vi "UHR-Fleezers Control (host) - 11.9c.vi"() -> ()   [LabVIEW 2014] (continued)
        n1081 = xnode "Read/Write Control"("FPGA VI Reference In"=w1450, "error in"=w1448, "Operating Mode"=w1447, "Operating Mode 2"=w1447, "Green FB On/Off"=w1446, "Red operating mode"=w1442, "RI operating mode 2"=w1442) -> ("error out"=w1449:errorcluster)  [unwired: 1 out]
      }
      event "Green Laser ON/OFF": Value Change {
        n1082 = event-data() -> ()  [unwired: 7 out]
        n1083 = property on="Green ON/Interlacing" class="Bool (strict)"("Val(Sgnl)"="Green Laser ON/OFF") -> ()  [unwired: 2 in, 2 out]
      }
      event "Test ttrig": Value Change {
        n1084 = event-data() -> ()  [unwired: 7 out]
        n1085 = xnode "Read/Write Control"("FPGA VI Reference In"=w1467, "error in"=w1466, "TTrig?"=TRUE) -> ("error out"=w1465:errorcluster)  [unwired: 1 out]
      }
      event "Neg. TTrig FPGA": Value Change {
        n1086 = event-data() -> ()  [unwired: 7 out]
        n1087 = xnode "Read/Write Control"("FPGA VI Reference In"=w1471, "error in"=w1470, "TTrig Negate Pos"="Neg. TTrig FPGA") -> ()  [unwired: 2 out]
      }
      event "- phase (APD 1 Gate)", "+ phase (APD 1 Gate)": Value Change {
        n1088 = event-data() -> ()  [unwired: 7 out]
        n1089 = local read "Phase Adj. (APD 1 Gate)"() -> (w1472:i16)
        n1090 = Negate(x=w1472) -> (-x=w1480:i16)
        n1091 = Select(t=w1480, s="- phase (APD 1 Gate)", f=w1472) -> (s? t:f=w1479:i16)
        n1092 = Or(x="- phase (APD 1 Gate)", y="+ phase (APD 1 Gate)") -> (x .or. y?=w1475:bool)
        n1093 = xnode "Read/Write Control"("FPGA VI Reference In"=w1482, "error in"=w1481, "Phase count adjustment (APD 1 Gate)"=w1479) -> ("FPGA VI Reference Out"=w1477:T20, "error out"=w1478:errorcluster)
        n1094 = xnode "Read/Write Control"("FPGA VI Reference In"=w1477, "error in"=w1478, "+ phase (APD 1 Gate)"=w1475) -> ("error out"=w1476:errorcluster)  [unwired: 1 out]
      }
      event "+ phase (APD 2 Gate)", "- phase (APD 2 Gate)": Value Change {
        n1095 = event-data() -> ()  [unwired: 7 out]
        n1096 = local read "Phase Adj. (APD 2 Gate)"() -> (w1483:i16)
        n1097 = Negate(x=w1483) -> (-x=w1491:i16)
        n1098 = Select(t=w1491, s="- phase (APD 2 Gate)", f=w1483) -> (s? t:f=w1490:i16)
        n1099 = Or(x="- phase (APD 2 Gate)", y="+ phase (APD 2 Gate)") -> (x .or. y?=w1486:bool)
        n1100 = xnode "Read/Write Control"("FPGA VI Reference In"=w1493, "error in"=w1492, "Phase count adjustment (APD 2 Gate)"=w1490) -> ("FPGA VI Reference Out"=w1488:T20, "error out"=w1489:errorcluster)
        n1101 = xnode "Read/Write Control"("FPGA VI Reference In"=w1488, "error in"=w1489, "+ phase (APD 2 Gate)"=w1486) -> ("error out"=w1487:errorcluster)  [unwired: 1 out]
      }
      event "Phase Adj. (APD Acq)", "+ phase (APD Acq)", "- phase (APD Acq)": Value Change {
        n1102 = event-data() -> ()  [unwired: 7 out]
        n1103 = local read "Phase Adj. (APD Acq)"() -> (w1496:i16)
        n1104 = Negate(x=w1496) -> (-x=w1502:i16)
        n1105 = Select(t=w1502, s="+ phase (APD Acq)", f=w1496) -> (s? t:f=w1501:i16)
        n1106 = Or(x="+ phase (APD Acq)", y="- phase (APD Acq)") -> (x .or. y?=w1497:bool)
        n1107 = xnode "Read/Write Control"("FPGA VI Reference In"=w1504, "error in"=w1503, "Phase Count Adjustment (APD Acq)"=w1501) -> ("FPGA VI Reference Out"=w1499:T20, "error out"=w1500:errorcluster)
        n1108 = xnode "Read/Write Control"("FPGA VI Reference In"=w1499, "error in"=w1500, "+ phase (APD Acq)"=w1497) -> ("error out"=w1498:errorcluster)  [unwired: 1 out]
      }
      event "Phase adj. (GI)", "+ phase (GI)", "- phase (GI)", "+phase (RI)", "- phase (RI)", "Phase adj. (RI)": Value Change {
        n1109 = event-data() -> ()  [unwired: 7 out]
        n1110 = Negate(x="Phase adj. (GI)") -> (-x=w1519:i16)
        n1111 = Select(t=w1519, s="+ phase (GI)", f="Phase adj. (GI)") -> (s? t:f=w1518:i16)
        n1112 = Or(x="+ phase (GI)", y="- phase (GI)") -> (x .or. y?=w1514:bool)
        n1113 = Negate(x="Phase adj. (RI)") -> (-x=w1509:i16)
        n1114 = Select(t=w1509, s="+phase (RI)", f="Phase adj. (RI)") -> (s? t:f=w1506:i16)
        n1115 = Or(x="+phase (RI)", y="- phase (RI)") -> (x .or. y?=w1505:bool)
        n1116 = xnode "Read/Write Control"("FPGA VI Reference In"=w1521, "error in"=w1520, "Phase count adjustment (GI)"=w1518, "Phase count adjustment (RI)"=w1506) -> ("FPGA VI Reference Out"=w1516:T20, "error out"=w1517:errorcluster)
        n1117 = xnode "Read/Write Control"("FPGA VI Reference In"=w1516, "error in"=w1517, "+ phase (GI)"=w1514, "+ phase (RI)"=w1505) -> ("error out"=w1515:errorcluster)  [unwired: 1 out]
      }
      event "+ phase (GI) 2", "- phase (GI) 2": Value Change {
        n1118 = event-data() -> ()  [unwired: 7 out]
        n1119 = Negate(x="Phase adj. (GI) 2") -> (-x=w1530:i16)
        n1120 = Select(t=w1530, s="+ phase (GI) 2", f="Phase adj. (GI) 2") -> (s? t:f=w1529:i16)
        n1121 = Or(x="+ phase (GI) 2", y="- phase (GI) 2") -> (x .or. y?=w1525:bool)
        n1122 = xnode "Read/Write Control"("FPGA VI Reference In"=w1532, "error in"=w1531, "Phase count adjustment (GI) 2"=w1529) -> ("FPGA VI Reference Out"=w1527:T20, "error out"=w1528:errorcluster)
        n1123 = xnode "Read/Write Control"("FPGA VI Reference In"=w1527, "error in"=w1528, "+ phase (GI) 2"=w1525) -> ("error out"=w1526:errorcluster)  [unwired: 1 out]
      }
      event "Phase adj. (Green FB)", "- phase (Green FB)", "+ phase (Green FB)": Value Change {
        n1124 = event-data() -> ()  [unwired: 7 out]
        n1125 = Negate(x="Phase adj. (Green FB)") -> (-x=w1541:i16)
        n1126 = Select(t=w1541, s="+ phase (Green FB)", f="Phase adj. (Green FB)") -> (s? t:f=w1540:i16)
        n1127 = Or(x="+ phase (Green FB)", y="- phase (Green FB)") -> (x .or. y?=w1536:bool)
        n1128 = xnode "Read/Write Control"("FPGA VI Reference In"=w1543, "error in"=w1542, "Phase count adjustment (Green FB)"=w1540) -> ("FPGA VI Reference Out"=w1538:T20, "error out"=w1539:errorcluster)
        n1129 = xnode "Read/Write Control"("FPGA VI Reference In"=w1538, "error in"=w1539, "+ phase (Green FB)"=w1536) -> ("error out"=w1537:errorcluster)  [unwired: 1 out]
      }
      event "Invert APD Gate", "APD Gate ON Count", "APD Gate OFF Count", "APD Gate", "APD Integration Time (s)", "APD 1 AO Mult.", "APD 2 AO Mult.", "Duty frequency (ON 1/N cycles)": Value Change {
        n1130 = event-data() -> ()  [unwired: 7 out]
        n1131 = Add(x="Interlace ON count", y="Interlace OFF count") -> (x+y=w1547:u16)
        n1132 = Add(x="APD Gate ON Count", y="APD Gate OFF Count") -> (x+y=w1560:u16)
        n1133 = Multiply(x="Duty frequency (ON 1/N cycles)", y=w1547) -> (x*y=w1546:u16)
        "Green FB Count" <- w1546
        n1134 = Subtract(x=w1546, y="Interlace ON count") -> (x-y=w1544:u16)
        n1135 = Multiply(x=w1560, y="Duty frequency (ON 1/N cycles)") -> (x*y=w1559:u16)
        n1136 = Subtract(x=w1559, y="APD Gate ON Count") -> (x-y=w1558:u16)
        n1137 = local read "DMA Update Period (s)"() -> (w1561:dbl)
        n1138 = Multiply(x="APD Integration Time (s)", y=40000000.0) -> (x*y=w1566:dbl)
        n1139 = Reciprocal(x="APD Integration Time (s)") -> (1/x=→"APD Acq Rate (Hz)":dbl)
        n1140 = To Unsigned Long Integer(number=w1566) -> (unsigned 32bit integer=w1550:u32)
        "APD Int. Count" <- w1550
        n1141 = xnode "Read/Write Control"("FPGA VI Reference In"=w1570, "error in"=w1569, "Invert APD Gate"="Invert APD Gate", "APD Gate ON Count"="APD Gate ON Count", "APD Gate OFF Count"=w1558, "APD Acq Rate Count"=w1550, "APD Gate Operating Mode"="APD Gate", "APD 1 AO scale factor"="APD 1 AO Mult.", "APD 2 AO scale factor"="APD 2 AO Mult.", "Green interlace ON count"="Interlace ON count", "Green interlace OFF count"=w1544, "Green interlace ON count 2"="Interlace ON count", "Green interlace OFF count 2"=w1544, "Green FB Count"=w1546, "RI ON count"="Interlace ON count", "RI OFF count"=w1544) -> ("error out"=w1568:errorcluster)  [unwired: 1 out]
        n1142 = Divide(x=w1561, y="APD Integration Time (s)") -> (x/y=w1564:dbl)
        n1143 = Multiply(x=2.0, y=w1564) -> (x*y=w1563:dbl)
        n1144 = local write "APD Samples/FIFO Acq."(w1564) -> ()
        n1145 = local write "APD Elements/DMA read"(w1563) -> ()
      }
      event "Number of F/B Scans (AOD)", "Scan Speed (nm/s)", "Scan BD", "Initial D (MHz)", "Step Size (nm)", "Scan Range (nm)", "Wiggle amp 1 (units?)": Value Change {
        w1632 = 123.0  # AOM cal (nm/MHz)
        n1146 = event-data() -> ()  [unwired: 7 out]
        n1147 = local read "BD 1 Frequency 1 (MHz)"() -> (w1615:dbl)
        n1148 = local read "AOM X Cal (nm/MHz)"() -> (w1607:dbl)
        n1149 = local read "BD 2 Frequency 1 (MHz)"() -> (w1621:dbl)
        n1150 = local read "X RF Frequency Limits (MHz)"() -> (w1619:T17)
        n1151 = local read "Y RF Frequency Limits (MHz)"() -> (w1616:T17)
        n1152 = Negate(x="Scan Range (nm)") -> (-x=w1585:dbl)
        n1153 = Divide(x=w1585, y=w1607) -> (x/y=w1589:dbl)
        n1154 = Select(t=w1619, s="Scan BD", f=w1616) -> (s? t:f=w1618:T17)
        n1155 = Select(t=w1615, s="Scan BD", f=w1621) -> (s? t:f=w1620:dbl)
        n1156 = Unbundle By Name(w1618) -> ("Maximum"=w1627:dbl, "Minimum"=w1626:dbl)
        n1157 = Add(x=w1589, y=w1620) -> (x+y=w1624:dbl)
        n1158 = Divide(x=w1585, y="Step Size (nm)") -> (x/y=w1604:dbl)
        n1159 = Divide(x="Step Size (nm)", y=w1607) -> (x/y=w1613:dbl)
        n1160 = Absolute Value(x=w1604) -> (abs(x)=w1588:dbl)
        n1161 = Sign(1:w1585) -> (0:w1586:dbl)
        n1162 = In Range and Coerce(upper limit=w1627, x=w1624, lower limit=w1626) -> (coerced(x)=w1623:dbl, In Range?=w1625:bool)
        n1163 = To Unsigned Quad Integer(1:w1588) -> (0:w1603:u64)
        "Scan steps (AOD)" <- w1603
        n1164 = call "IR AOM freq to word.vi"("Frequency In (MHz)"=w1613) -> ("Frequency Word Out (double)"=w1610:dbl)
        n1165 = Multiply(x=w1586, y=w1610) -> (x*y=w1587:dbl)
        n1166 = Subtract(x=w1624, y=w1623) -> (x-y=w1622:dbl)
        n1167 = To Quad Integer(1:w1587) -> (0:w1609:i64)
        "Incr. int (AOD)" <- w1609
        n1168 = Subtract(x=w1589, y=w1622) -> (x-y=w1608:dbl)
        "Scan Range (MHz)" <- w1608
        n1169 = Select(t=w1589, s=w1625, f=w1608) -> (s? t:f=w1628:dbl)
        n1170 = Multiply(x=w1608, y=w1607) -> (x*y=w1606:dbl)
        n1171 = Decrement(x=w1603) -> (x-1=w1656:u64)
        n1172 = Negate(x=w1606) -> (-x=w1602:dbl)
        n1173 = local write "Scan Range (nm)"(w1602) -> ()
        n1174 = Divide(x=w1628, y=w1656) -> (x/y=w1612:dbl)
        "Scan Increment (MHz)" <- w1612
        n1175 = call "IR AOM freq to word.vi"("Frequency In (MHz)"=w1612) -> ("Frequency Word Out (double)"=w1611:dbl)
        n1176 = Divide(x="Step Size (nm)", y="Scan Speed (nm/s)") -> (x/y=w1599:dbl)
        n1177 = To Quad Integer(1:w1611) -> ()  [unwired: 1 out]
        n1178 = local read "Number Interlace Sets"() -> (w1583:u8)
        n1179 = local read "AI Count (ticks)"() -> (w1584:u32)
        n1180 = local read "Total Counts (ticks)"() -> (w1582:u32)
        n1181 = local read "# Samples/trap"() -> (w1614:u32)
        n1182 = Multiply(x=w1584, y=w1583) -> (x*y=w1581:u32)
        n1183 = Divide(x=w1582, y=w1581) -> (x/y=w1580:dbl)
        n1184 = Select(t=w1615, s="Scan BD", f=w1621) -> (s? t:f=w1653:dbl)
        "Initial freq. (MHz)" <- w1653
        n1185 = Add(x=w1628, y=w1653) -> (x+y=→"Final freq. (MHz)":dbl)
        n1186 = Divide(x=w1582, y=40000000.0) -> (x/y=w1598:dbl)
        n1187 = Divide(x=w1599, y=w1598) -> (x/y=w1597:dbl)
        n1188 = To Unsigned Quad Integer(1:w1597) -> (0:w1572:u64)
        n1189 = Quotient & Remainder(x=w1572, y=u64 2) -> (x-y*floor(x/y)=w1576:u64)  [unwired: 1 out]
        n1190 = Equal?(x=w1576, y=u64 0) -> (x = y?=w1574:bool)
        n1191 = Decrement(x=w1572) -> (x-1=w1573:u64)
        n1192 = Select(t=w1572, s=w1574, f=w1573) -> (s? t:f=w1571:u64)
        "Cycles/step (AOD)" <- w1571
        n1193 = xnode "Read/Write Control"("FPGA VI Reference In"=w1664, "error in"=w1663, "Scan steps"=w1603, "Number of scans"="Number of F/B Scans (AOD)", "Cycles per step"=w1571, "Scan freq.  increment"=w1609, "Scan BD"="Scan BD") -> ("error out"=w1662:errorcluster)  [unwired: 1 out]
        n1194 = Multiply(x=w1603, y=w1571) -> (x*y=w1657:u64)
        n1195 = Multiply(x=w1657, y=u64 2) -> (x*y=w1579:u64)
        n1196 = Multiply(x=w1580, y=w1579) -> (x*y=w1578:dbl)
        "Data points/scan (f/b)" <- w1578
        n1197 = Multiply(x=w1578, y="Number of F/B Scans (AOD)") -> (x*y=w1660:dbl)
        "Data points/scans" <- w1660
        n1198 = Divide(x=w1660, y=w1614) -> (x/y=→"N sets should be saved":dbl)
        n1199 = Multiply(x=w1657, y=w1598) -> (x*y=w1596:dbl)
        "Time/Scan (s) (AOD)" <- w1596
        n1200 = Select(t=w1628, s="Scan BD", f=0.0) -> (s? t:f=w1654:dbl)
        n1201 = Select(t=0.0, s="Scan BD", f=w1628) -> (s? t:f=w1650:dbl)
        n1202 = local read "BD 2 Frequency 2 (MHz)"() -> (w1646:dbl)
        n1203 = local read "BD 1 Frequency 2 (MHz)"() -> (w1649:dbl)
        n1204 = Add(x=w1650, y=w1621) -> (x+y=w1647:dbl)
        n1205 = Add(x=w1615, y=w1654) -> (x+y=w1648:dbl)
        n1206 = Multiply(x=w1596, y=2.0) -> (x*y=w1595:dbl)
        n1207 = Multiply(x=w1595, y="Number of F/B Scans (AOD)") -> (x*y=w1592:dbl)
        n1208 = Divide(x=w1592, y=60.0) -> (x/y=→"Time to Finish All (min)":dbl)
        n1209 = Add(x="Trap 2 Bead Size (nm)", y="Trap 1 Bead Size (nm)") -> (x+y=w1636:dbl)
        n1210 = Divide(x=w1636, y=2.0) -> (x/y=w1630:dbl)
        n1211 = Subtract(x=w1647, y=w1646) -> (x-y=w1644:dbl)
        n1212 = Subtract(x=w1648, y=w1649) -> (x-y=w1645:dbl)
        n1213 = local read "Initial D (MHz)"() -> (w1633:dbl)
        n1214 = Square(x=w1644) -> (x^2=w1643:dbl)
        n1215 = Square(x=w1645) -> (x^2=w1642:dbl)
        n1216 = Add(x=w1642, y=w1643) -> (x+y=w1641:dbl)
        n1217 = Square Root(x=w1641) -> (sqrt(x)=w1640:dbl)
        "Final D (MHz)" <- w1640
        n1218 = Multiply(x=w1632, y=w1640) -> (x*y=w1639:dbl)
        n1219 = Multiply(x=w1633, y=w1632) -> (x*y=w1631:dbl)
        n1220 = Subtract(x=w1631, y=w1630) -> (x-y=→"Initial sep (nm)":dbl)
        n1221 = Subtract(x=w1639, y=w1630) -> (x-y=→"Final sep (nm)":dbl)
      }
      event "Freq or Amp switch first", "Swap F1 and F2", "Freq switch delay", "Amp switch delay": Value Change {
        n1222 = event-data() -> ()  [unwired: 7 out]
        n1223 = local read "Freq or Amp switch first"() -> (w1665:bool)
        n1224 = local read "Amp switch delay"() -> (w1666:u16)
        n1225 = local read "Freq switch delay"() -> (w1668:u16)
        n1226 = local read "Swap F1 and F2"() -> (w1667:bool)
        n1227 = xnode "Read/Write Control"("FPGA VI Reference In"=w1671, "error in"=w1670, "Freq switch delay"=w1668, "Swap F1 and F2"=w1667, "Amp switch delay"=w1666, "Freq or Amp switch first"=w1665) -> ("error out"=w1669:errorcluster)  [unwired: 1 out]
      }
      event "Scan steps (MCL)", "Number of scans (MCL)", "Scan Range (V)\n(of steps)", "2D or 1D Scan", "N APD Samp/step", "Fast Scan Dir", "Continuous MCL Scanning", "Scan lines (y)": Value Change {
        w1673 = 32767.0 ("y")
        n1228 = event-data() -> ()  [unwired: 7 out]
        n1229 = Select(t="Scan lines (y)", s="2D or 1D Scan", f="Number of scans (MCL)") -> (s? t:f=w1678:u64)
        n1230 = Decrement(x="Scan steps (MCL)") -> (x-1=w1694:u64)
        n1231 = Divide(x="Scan Range (V)\n(of steps)", y=w1694) -> (x/y=w1693:dbl)
        "Desired Scan Incr (V)" <- w1693
        n1232 = local read "APD Integration Time (s)"() -> (w1686:dbl)
        n1233 = Multiply(x=w1693, y=w1673) -> (x*y=w1702:dbl)
        n1234 = Divide(x=w1702, y=10.0) -> (x/y=w1692:dbl)
        "Desired incr (int)" <- w1692
        n1235 = local read "Update Count (MCL)"() -> (w1698:u32)
        n1236 = Round Toward -Infinity(1:w1692) -> (0:w1701:dbl)
        n1237 = To Word Integer(number=w1701) -> (16bit integer=w1676:i16)
        "Actual Incr. int (MCL)" <- w1676
        n1238 = Multiply(x=w1686, y=40000000.0) -> (x*y=w1699:dbl)
        n1239 = Divide(x=w1699, y=w1698) -> (x/y=w1697:dbl)
        n1240 = Multiply(x=i16 10, y=w1676) -> (x*y=w1674:i16)
        n1241 = Multiply(x="N APD Samp/step", y=w1697) -> (x*y=w1696:dbl)
        "Cycles/step (MCL)" <- w1696
        n1242 = Divide(x=w1674, y=w1673) -> (x/y=→"Actual MCL Inc (V)":dbl)
        n1243 = Multiply(x="N APD Samp/step", y="Scan steps (MCL)") -> (x*y=w1688:dbl)
        n1244 = local read "APD Samples/FIFO Acq."() -> (w1685:dbl)
        n1245 = Multiply(x=w1688, y=u64 2) -> (x*y=w1687:dbl)
        "Data points/scan (f+b)" <- w1687
        n1246 = Multiply(x=w1687, y=w1678) -> (x*y=w1705:dbl)
        "Data points/scans (MCL)" <- w1705
        n1247 = Multiply(x=w1686, y=w1687) -> (x*y=w1679:dbl)
        "Time/f+b scan (s) (MCL)" <- w1679
        n1248 = Divide(x=w1705, y=w1685) -> (x/y=→"N sets should be saved (MCL)":dbl)
        n1249 = Multiply(x=w1679, y=w1678) -> (x*y=→"Total Time (s)":dbl)
        n1250 = Not(x="Fast Scan Dir") -> (.not. x?=w1683:bool)
        n1251 = xnode "Read/Write Control"("FPGA VI Reference In"=w1709, "error in"=w1708, "Scan steps (MCL)"="Scan steps (MCL)", "Number of scans (MCL)"=w1678, "Cycles per step (MCL)"=w1696, "Scan freq.  increment (MCL)"=w1676, "1D or 2D Scan?"="2D or 1D Scan", "MCL Scan Axis"=w1683, "Cont. Scan (MCL)"="Continuous MCL Scanning") -> ("error out"=w1707:errorcluster)  [unwired: 1 out]
      }
      event "Read Cal": Value Change {
        w1711 = 1000.0 ("y")
        n1252 = event-data() -> ()  [unwired: 7 out]
        n1253 = local read "Save file name"() -> (w1736:path)
        n1254 = local write "Read Cal"(FALSE ("Read Cal")) -> ()
        n1255 = Strip Path(path=w1736) -> (stripped path=w1735:path)  [unwired: 1 out]
        n1256 = Path To String(path=w1735) -> (string=w1734:string)
        n1257 = Concatenate Strings(w1734, "\\current.cal" ("string")) -> (w1732:string)
        n1258 = String To Path(string=w1732) -> (path=w1731:path)
        n1259 = Open/Create/Replace File(file path (use dialog)=w1731, operation (0:open)=T26."open", access (0:read/write)=enum16{"read/write", "read-only", "write-only"}."read-only") -> (refnum out=w1739:refnum<file>, error out=w1725:errorcluster)  [unwired: 1 in, 3 out]
        n1260 = Deny Access(4:w1725, 7:w1739) -> (0:w1724:errorcluster, 3:w1730:refnum<file>)  [unwired: 1 out]
        n1261 = Read from Binary File(5:0.0, 8:w1724, 9:T25."big-endian, network order" ("byte order (0:big-endian, network order)"), 10:-1 ("count (1)"), 11:w1730) -> (0:w1723:errorcluster, 2:w1721:dbl[], 3:w1726:refnum<file>)  [unwired: 2 out]
        n1262 = Array To Cluster(array=w1721) -> (cluster=w1720:T28)
        n1263 = Unbundle(w1720) -> ("[0]"=w1719:dbl, "[1]"=w1718:dbl, "[2]"=w1717:dbl, "[3]"=w1716:dbl, "[4]"=w1715:dbl, "[5]"=w1714:dbl)
        n1264 = Close File(refnum=w1726, error in=w1723) -> (error out=→"Read cal error":errorcluster)  [unwired: 1 out]
        n1265 = Multiply(x=w1714, y=w1711) -> (x*y=w1712:dbl)
        n1266 = local write "T2 k_x (pN/nm)"(w1716) -> ()
        n1267 = local write "T1 k_x (pN/nm)"(w1717) -> ()
        n1268 = local write "T1 a_x (nm/V)"(w1719) -> ()
        n1269 = local write "T2 a_x (nm/V)"(w1718) -> ()
        n1270 = Multiply(x=w1715, y=w1711) -> (x*y=w1713:dbl)
        n1271 = local write "T1 offset_x (mV)"(w1713) -> ()
        n1272 = local write "T2 offset_x (mV)"(w1712) -> ()
      }
      event "Read FX file": Value Change {
        n1273 = event-data() -> ()  [unwired: 7 out]
        n1274 = local write "Read FX file"(FALSE ("Read residual")) -> ()
        n1275 = local read "Save file name"() -> (w1764:path)
        n1276 = Strip Path(path=w1764) -> (stripped path=w1763:path)  [unwired: 1 out]
        n1277 = Path To String(path=w1763) -> (string=w1762:string)
        n1278 = Concatenate Strings(w1762, "\\current.cal" ("string")) -> (w1760:string)
        n1279 = String To Path(string=w1760) -> (path=w1759:path)
        n1280 = Open/Create/Replace File(file path (use dialog)=w1759, operation (0:open)=T26."open", access (0:read/write)=enum16{"read/write", "read-only", "write-only"}."read-only") -> (refnum out=w1756:refnum<file>, error out=w1753:errorcluster)  [unwired: 3 in, 1 out]
        n1281 = Deny Access(4:w1753, 7:w1756) -> (0:w1752:errorcluster, 3:w1755:refnum<file>)  [unwired: 1 in]
        n1282 = Read from Binary File(5:0.0, 8:w1752, 9:T25."big-endian, network order" ("byte order (0:big-endian, network order)"), 10:-1 ("count"), 11:w1755) -> (0:w1748:errorcluster, 2:w1742:dbl[], 3:w1749:refnum<file>)  [unwired: 1 in, 1 out]
        n1283 = Index Array(array=w1742, index=6) -> (element=→"Bad fit error":dbl)
        n1284 = Index Array(array=w1742, index=7) -> (element=→"Fit offset":dbl)
        n1285 = Index Array(array=w1742, index=8) -> (element=→"Hyst. error":dbl)
        n1286 = Close File(refnum=w1749, error in=w1748) -> ()  [unwired: 2 out]
      }
      event "Abort MCL Scan": Value Change {
        n1287 = event-data() -> ()  [unwired: 7 out]
        n1288 = local write "MCL Scanning"(FALSE ("MCL Scanning")) -> ()
        n1289 = xnode "Read/Write Control"("FPGA VI Reference In"=w1769, "error in"=w1768, "Abort scan (MCL)"="Abort MCL Scan") -> ("error out"=w1767:errorcluster)  [unwired: 1 out]
      }
      event "Update Count (MCL)": Value Change {
        n1290 = event-data() -> ()  [unwired: 7 out]
        n1291 = xnode "Read/Write Control"("FPGA VI Reference In"=w1773, "error in"=w1772, "MCL count"="Update Count (MCL)") -> ("error out"=w1771:errorcluster)  [unwired: 1 out]
      }
      event "Phase adjust (MCL)", "+ phase (MCL)", "- phase (MCL)": Value Change {
        n1292 = event-data() -> ()  [unwired: 7 out]
        n1293 = Negate(x="Phase adjust (MCL)") -> (-x=w1782:i16)
        n1294 = Select(t=w1782, s="- phase (MCL)", f="Phase adjust (MCL)") -> (s? t:f=w1780:i16)
        n1295 = Or(x="- phase (MCL)", y="+ phase (MCL)") -> (x .or. y?=w1775:bool)
        n1296 = xnode "Read/Write Control"("FPGA VI Reference In"=w1784, "error in"=w1783, "Phase count adjustment (MCL)"=w1780) -> ("FPGA VI Reference Out"=w1776:T20, "error out"=w1777:errorcluster)
        n1297 = xnode "Read/Write Control"("FPGA VI Reference In"=w1776, "error in"=w1777, "+ phase (MCL)"=w1775) -> ("error out"=w1774:errorcluster)  [unwired: 1 out]
      }
      event "Abort AOD Scan": Value Change {
        n1298 = event-data() -> ()  [unwired: 7 out]
        n1299 = xnode "Read/Write Control"("FPGA VI Reference In"=w1788, "error in"=w1787, "Abort scan"="Abort AOD Scan") -> ("error out"=w1786:errorcluster)  [unwired: 1 out]
      }
      event "Continuous AOD Scanning": Value Change {
        n1300 = event-data() -> ()  [unwired: 7 out]
        n1301 = xnode "Read/Write Control"("FPGA VI Reference In"=w1792, "error in"=w1791, "Cont. Scan"="Continuous AOD Scanning") -> ("error out"=w1790:errorcluster)  [unwired: 1 out]
      }
      event "Index": Value Change {
        n1302 = event-data() -> ()  [unwired: 7 out]
        n1303 = call "Create new save file.vi"("Insert"="", "Ext"=".dat" ("string"), "Index In"="Index") -> ("Path Out"=→"Save file name":path, "Index Out"=w1793:dbl)
        "Save index" <- w1793
        n1304 = local write "Index"(w1793) -> ()
      }
      event "AO1", "AO2": Value Change {
        w1808 = 10.0 ("y")
        w1807 = 32767.0 ("y")
        n1305 = event-data() -> ()  [unwired: 7 out]
        n1306 = local read "AO2"() -> (w1806:dbl)
        n1307 = local read "AO1"() -> (w1803:dbl)
        n1308 = Multiply(x=w1803, y=w1807) -> (x*y=w1802:dbl)
        n1309 = Multiply(x=w1806, y=w1807) -> (x*y=w1805:dbl)
        n1310 = Divide(x=w1802, y=w1808) -> (x/y=w1801:dbl)
        n1311 = Divide(x=w1805, y=w1808) -> (x/y=w1804:dbl)
        n1312 = To Word Integer(number=w1801) -> (16bit integer=w1809:i16)
        n1313 = To Word Integer(number=w1804) -> (16bit integer=w1810:i16)
        n1314 = xnode "Read/Write Control"("FPGA VI Reference In"=w1800, "error in"=w1799, "AO1"=w1809, "AO2"=w1810) -> ("error out"=w1798:errorcluster)  [unwired: 1 out]
      }
      event "Inject Pump 1": Value Change {
        n1315 = event-data() -> ()  [unwired: 7 out]
        n1316 = local read "Use Harvard pumps\nfor beads (else Chemyx)"() -> (w1812:bool)
        n1317 = case shown="True" w1812 {
          tunnel: "Inject Pump 1" -> [w1816 w1854]
          tunnel: w1811 -> [_ w1855]
          frame False {
            n1318 = local read "Pump write delay (ms)"() -> (w1815:dbl)
            n1319 = local read "Chemyx Syringe Pump Serial Port"() -> (w1814:refnum<visa-resource-name>)
            n1320 = case shown="True" w1816 {
              tunnel: w1815 -> [w1822 w1836]
              tunnel: w1814 -> [w1819 w1835]
              frame False {
                n1321 = flat-sequence {
                  tunnel: w1819 -> [w1823]
                  tunnel: [w1823] -> w1820
                  tunnel: w1822 -> [_]
                  tunnel: [w1826] -> w1821
                  tunnel: w1820 -> [w1826]
                  tunnel: w1821 -> [w1827]
                  tunnel: [w1827] -> w1817
                  tunnel: [w1829] -> w1818
                  tunnel: w1817 -> [w1829]
                  tunnel: w1818 -> [w1831]
                  frame #0 {
                    n1322 = call "Write to pump.vi"("string"="enter pump1", "VISA resource name"=w1823) -> ()  [unwired: 1 out]
                  }
                  frame #1 {
                    n1323 = Wait (ms)(milliseconds to wait="Pump pause delay (ms)") -> ()  [unwired: 1 out]
                  }
                  frame #2 {
                    n1324 = call "Write to pump.vi"("string"="stop", "VISA resource name"=w1827) -> ()  [unwired: 1 out]
                  }
                  frame #3 {
                    n1325 = Wait (ms)(milliseconds to wait=u32 500) -> ()  [unwired: 1 out]
                  }
                  frame #4 {
                    n1326 = call "Write to pump.vi"("string"="stop", "VISA resource name"=w1831) -> ()  [unwired: 1 out]
                  }
                }
              }
              frame True {
                n1327 = flat-sequence {
                  tunnel: w1835 -> [w1845]
                  tunnel: w1836 -> [w1840]
                  tunnel: w1836 -> [w1847]
                  tunnel: w1835 -> [w1848]
                  tunnel: [w1848] -> w1833
                  tunnel: [w1850] -> w1834
                  tunnel: w1833 -> [w1850]
                  tunnel: w1834 -> [w1852]
                  frame #0 {
                    n1328 = local read "All Pump Parameters"() -> (w1839:T5)
                    n1329 = Unbundle By Name(w1839) -> ("Pump 1"=w1846:T29)
                    n1330 = call "Set pump parameters.vi"("Pump write delay (ms)"=w1840, "Volume (uL)"="Ch 1 Inject Volume (uL)", "Rate (uL/h)"="Ch 1 Inject Rate (ul/h)", "Units"=4.0, "Pump #"=1.0, "Pump Parameters In"=w1846, "VISA resource name"=w1845) -> ("Pump Parameters Out"=w1838:T29)  [unwired: 3 in]
                    n1331 = Bundle By Name(cluster=w1839, "Pump 1"=w1838) -> (w1837:T5)
                    n1332 = local write "All Pump Parameters"(w1837) -> ()
                  }
                  frame #1 {
                    n1333 = Wait (ms)(milliseconds to wait=w1847) -> ()  [unwired: 1 out]
                  }
                  frame #2 {
                    n1334 = call "Write to pump.vi"("string"="start", "VISA resource name"=w1848) -> ()  [unwired: 1 out]
                  }
                  frame #3 {
                    n1335 = Wait (ms)(milliseconds to wait=u32 500) -> ()  [unwired: 1 out]
                  }
                  frame #4 {
                    n1336 = call "Write to pump.vi"("string"="start", "VISA resource name"=w1852) -> ()  [unwired: 1 out]
                  }
                }
              }
            }
          }
          frame True {
            n1337 = case shown="True" w1854 {
              tunnel: w1855 -> [w1856 w1866]
              frame False {
                n1338 = flat-sequence {
                  tunnel: w1856 -> [w1858]
                  frame #0 {
                    n1339 = local write "Flushing P1"(FALSE ("Flushing P1")) -> ()
                    n1340 = Concatenate Strings("stop" ("string"), "\r") -> (w1860:string)
                    n1341 = VISA Write(VISA resource name=w1858, write buffer=w1860) -> ()  [unwired: 1 in, 3 out]
                  }
                  frame #1 {
                    n1342 = property on="Clear Volume P1" class="Bool (strict)"("Val(Sgnl)"=TRUE ("Value (Signaling)")) -> ()  [unwired: 2 in, 2 out]
                  }
                }
              }
              frame True {
                n1343 = local read "Normal Flow Rate (ul/h) P1"() -> (w1864:dbl)
                n1344 = Number To Decimal String(number=w1864) -> (decimal integer string=w1870:string)  [unwired: 1 in]
                n1345 = Concatenate Strings("irate  " ("string"), w1870, " u/h" ("string"), "\r") -> (w1868:string)
                n1346 = VISA Write(VISA resource name=w1866, write buffer=w1868) -> (VISA resource name out=w1865:refnum<visa-resource-name>)  [unwired: 1 in, 2 out]
                n1347 = Concatenate Strings("irun" ("string"), "\r") -> (w1872:string)
                n1348 = VISA Write(VISA resource name=w1865, write buffer=w1872) -> ()  [unwired: 1 in, 3 out]
              }
            }
          }
        }
      }
      event "Inject Pump 3": Value Change {
        n1349 = event-data() -> ()  [unwired: 7 out]
        n1350 = local read "Use Harvard pumps\nfor beads (else Chemyx)"() -> (w1875:bool)
        n1351 = case shown="True" w1875 {
          tunnel: "Inject Pump 3" -> [w1879 w1918]
          tunnel: w1874 -> [_ w1917]
          frame False {
            n1352 = local read "Pump write delay (ms)"() -> (w1878:dbl)
            n1353 = case shown="True" w1879 {
              tunnel: w1878 -> [w1885 w1899]
              tunnel: "Chemyx Syringe Pump Serial Port" -> [w1882 w1898]
              frame False {
                n1354 = flat-sequence {
                  tunnel: w1882 -> [w1886]
                  tunnel: [w1886] -> w1883
                  tunnel: w1885 -> [_]
                  tunnel: [w1889] -> w1884
                  tunnel: w1883 -> [w1889]
                  tunnel: w1884 -> [w1890]
                  tunnel: [w1890] -> w1880
                  tunnel: [w1892] -> w1881
                  tunnel: w1880 -> [w1892]
                  tunnel: w1881 -> [w1894]
                  frame #0 {
                    n1355 = call "Write to pump.vi"("string"="enter pump3", "VISA resource name"=w1886) -> ()  [unwired: 1 out]
                  }
                  frame #1 {
                    n1356 = local read "Pump pause delay (ms)"() -> (w1888:u32)
                    n1357 = Wait (ms)(milliseconds to wait=w1888) -> ()  [unwired: 1 out]
                  }
                  frame #2 {
                    n1358 = call "Write to pump.vi"("string"="stop", "VISA resource name"=w1890) -> ()  [unwired: 1 out]
                  }
                  frame #3 {
                    n1359 = Wait (ms)(milliseconds to wait=u32 0) -> ()  [unwired: 1 out]
                  }
                  frame #4 {
                    n1360 = call "Write to pump.vi"("string"="stop", "VISA resource name"=w1894) -> ()  [unwired: 1 out]
                  }
                }
              }
              frame True {
                n1361 = flat-sequence {
                  tunnel: w1898 -> [w1908]
                  tunnel: w1899 -> [w1903]
                  tunnel: w1899 -> [w1910]
                  tunnel: w1898 -> [w1911]
                  tunnel: [w1911] -> w1897
                  tunnel: [w1914] -> w1896
                  tunnel: w1897 -> [w1914]
                  tunnel: w1896 -> [w1915]
                  frame #0 {
                    n1362 = local read "All Pump Parameters"() -> (w1902:T5)
                    n1363 = Unbundle By Name(w1902) -> ("Pump 3"=w1909:T29)
                    n1364 = call "Set pump parameters.vi"("Pump write delay (ms)"=w1903, "Volume (uL)"="Ch 3 Inject Volume (uL)", "Rate (uL/h)"="Ch 3 Inject Rate (ul/h)", "Units"=4.0, "Pump #"=3.0, "Pump Parameters In"=w1909, "VISA resource name"=w1908) -> ("Pump Parameters Out"=w1901:T29)  [unwired: 3 in]
                    n1365 = Bundle By Name(cluster=w1902, "Pump 3"=w1901) -> (w1900:T5)
                    n1366 = local write "All Pump Parameters"(w1900) -> ()
                  }
                  frame #1 {
                    n1367 = Wait (ms)(milliseconds to wait=w1910) -> ()  [unwired: 1 out]
                  }
                  frame #2 {
                    n1368 = call "Write to pump.vi"("string"="start", "VISA resource name"=w1911) -> ()  [unwired: 1 out]
                  }
                  frame #3 {
                    n1369 = Wait (ms)(milliseconds to wait=u32 500) -> ()  [unwired: 1 out]
                  }
                  frame #4 {
                    n1370 = call "Write to pump.vi"("string"="start", "VISA resource name"=w1915) -> ()  [unwired: 1 out]
                  }
                }
              }
            }
          }
          frame True {
            n1371 = case shown="True" w1918 {
              tunnel: w1917 -> [w1919 w1926]
              frame False {
                n1372 = flat-sequence {
                  tunnel: w1919 -> [w1921]
                  frame #0 {
                    n1373 = local write "Flushing P3"(FALSE ("Flushing P3")) -> ()
                    n1374 = Concatenate Strings("stop" ("string"), "\r") -> (w1923:string)
                    n1375 = VISA Write(VISA resource name=w1921, write buffer=w1923) -> ()  [unwired: 1 in, 3 out]
                  }
                  frame #1 {
                    n1376 = property on="Clear Volume P3" class="Bool (strict)"("Val(Sgnl)"=TRUE ("Value (Signaling)")) -> ()  [unwired: 2 in, 2 out]
                  }
                }
              }
              frame True {
                n1377 = local read "Normal Flow Rate (ul/h) P3"() -> (w1927:dbl)
                n1378 = Number To Decimal String(number=w1927) -> (decimal integer string=w1933:string)  [unwired: 1 in]
                n1379 = Concatenate Strings("irate  " ("string"), w1933, " u/h" ("string"), "\r") -> (w1931:string)
                n1380 = VISA Write(VISA resource name=w1926, write buffer=w1931) -> (VISA resource name out=w1929:refnum<visa-resource-name>)  [unwired: 1 in, 2 out]
                n1381 = Concatenate Strings("irun" ("string"), "\r") -> (w1935:string)
                n1382 = VISA Write(VISA resource name=w1929, write buffer=w1935) -> ()  [unwired: 1 in, 3 out]
              }
            }
          }
        }
      }
      event "Inject Pump 2": Value Change {
        n1383 = event-data() -> ()  [unwired: 7 out]
        n1384 = local read "Pump write delay (ms)"() -> (w1939:dbl)
        n1385 = local read "Chemyx Syringe Pump Serial Port"() -> (w1937:refnum<visa-resource-name>)
        n1386 = flat-sequence {
          tunnel: w1937 -> [w1952]
          tunnel: w1939 -> [w1948]
          tunnel: "Inject Pump 2" -> [_]
          tunnel: w1939 -> [w1954]
          tunnel: w1937 -> [w1955]
          frame #0 {
            n1387 = local read "All Pump Parameters"() -> (w1947:T5)
            n1388 = Multiply(x=60.0, y="Flush Center Ch Rate (ul/m)") -> (x*y=w1944:dbl)
            n1389 = Unbundle By Name(w1947) -> ("Pump 2"=w1953:T29)
            n1390 = call "Set pump parameters.vi"("Pump write delay (ms)"=w1948, "Volume (uL)"="Flush Center Ch Volume (uL)", "Rate (uL/h)"=w1944, "Units"=3.0, "Pump #"=2.0, "Pump Parameters In"=w1953, "VISA resource name"=w1952) -> ("Pump Parameters Out"=w1946:T29)  [unwired: 3 in]
            n1391 = Bundle By Name(cluster=w1947, "Pump 2"=w1946) -> (w1945:T5)
            n1392 = Add(x="Flush Center Ch Volume (uL)", y="Total Volume\nFlushed (uL)") -> (x+y=w1941:dbl)
            n1393 = local write "All Pump Parameters"(w1945) -> ()
            n1394 = local write "Total Volume\nFlushed (uL)"(w1941) -> ()
          }
          frame #1 {
            n1395 = Wait (ms)(milliseconds to wait=w1954) -> ()  [unwired: 1 out]
          }
          frame #2 {
            n1396 = call "Write to pump.vi"("string"="start", "VISA resource name"=w1955) -> ()  [unwired: 1 out]
          }
        }
      }
      event "Sample Channel\nFlow": Value Change {
        n1397 = event-data() -> ()  [unwired: 7 out]
        n1398 = case shown="True" "Sample Channel\nFlow" {
          tunnel: w1958 -> [w1959 w1965]
          frame False {
            n1399 = flat-sequence {
              tunnel: w1959 -> [w1961]
              frame #0 {
                n1400 = local write "Flushing samp"(FALSE ("Flushing samp")) -> ()
                n1401 = Concatenate Strings("stop" ("string"), "\r") -> (w1964:string)
                n1402 = VISA Write(VISA resource name=w1961, write buffer=w1964) -> ()  [unwired: 1 in, 3 out]
              }
            }
          }
          frame True {
            n1403 = local read "Normal Flow rate (mL/h)"() -> (w1975:dbl)
            n1404 = Number To Decimal String(number=w1975) -> (decimal integer string=w1974:string)  [unwired: 1 in]
            n1405 = Concatenate Strings("irate " ("string"), w1974, " u/h" ("string"), "\r") -> (w1970:string)
            n1406 = VISA Write(VISA resource name=w1965, write buffer=w1970) -> (VISA resource name out=w1969:refnum<visa-resource-name>)  [unwired: 1 in, 2 out]
            n1407 = Concatenate Strings("irun" ("string"), "\r") -> (w1966:string)
            n1408 = VISA Write(VISA resource name=w1969, write buffer=w1966) -> ()  [unwired: 1 in, 3 out]
          }
        }
      }
      event "Start Flow": Value Change {
        n1409 = event-data() -> ()  [unwired: 7 out]
        n1410 = local write "Sample Channel\nFlow"(TRUE ("Sample Channel\nFlow")) -> ()
        n1411 = local write "Start Flow"(FALSE ("Start Flow")) -> ()
        n1412 = Concatenate Strings("irun" ("string"), "\r") -> (w1980:string)
        n1413 = VISA Write(VISA resource name=w1976, write buffer=w1980) -> ()  [unwired: 1 in, 3 out]
      }
      event "Stop Flow": Value Change {
        w1982 = FALSE ("Stop Flow")
        n1414 = event-data() -> ()  [unwired: 7 out]
        n1415 = local write "Stop Flow"(w1982) -> ()
        n1416 = local write "Sample Channel\nFlow"(w1982) -> ()
        n1417 = Concatenate Strings("stop" ("string"), "\r") -> (w1985:string)
        n1418 = VISA Write(VISA resource name=w1983, write buffer=w1985) -> ()  [unwired: 1 in, 3 out]
      }
      event "Normal Flow rate (mL/h)": Value Change {
        n1419 = event-data() -> ()  [unwired: 7 out]
        n1420 = Number To Decimal String(number="Normal Flow rate (mL/h)") -> (decimal integer string=w1992:string)  [unwired: 1 in]
        n1421 = Concatenate Strings("irate  " ("string"), w1992, " u/h" ("string"), "\r") -> (w1991:string)
        n1422 = VISA Write(VISA resource name=w1988, write buffer=w1991) -> ()  [unwired: 1 in, 3 out]
      }
      event "Flush Sample": Value Change {
        n1423 = event-data() -> ()  [unwired: 7 out]
        n1424 = flat-sequence {
          tunnel: w1994 -> [w2022]
          frame #0 {
            # "set parameters (rate, volume) for flush, clear volume"
            n1425 = Number To Decimal String(number="Flush rate (mL/m)") -> (decimal integer string=w2018:string)  [unwired: 1 in]
            n1426 = local write "Sample Channel\nFlow"(TRUE ("Sample Channel\nFlow")) -> ()
            n1427 = Concatenate Strings("irate  " ("string"), w2018, " u/m" ("string"), "\r") -> (w2020:string)
            n1428 = VISA Write(VISA resource name=w2022, write buffer=w2020) -> (VISA resource name out=w2016:refnum<visa-resource-name>)  [unwired: 1 in, 2 out]
            n1429 = Number To Decimal String(number="Flush volume (mL)") -> (decimal integer string=w2007:string)  [unwired: 1 in]
            n1430 = Reciprocal(x="Flush rate (mL/m)") -> (1/x=w2001:dbl)
            n1431 = Concatenate Strings("tvolume  " ("string"), w2007, " u" ("string"), "\r") -> (w2005:string)
            n1432 = Multiply(x=w2001, y="Flush volume (mL)") -> (x*y=w1999:dbl)
            n1433 = VISA Write(VISA resource name=w2016, write buffer=w2005) -> (VISA resource name out=w2004:refnum<visa-resource-name>)  [unwired: 1 in, 2 out]
            n1434 = Multiply(x=w1999, y=60.0) -> (x*y=→"Samp Flush Time (s)":dbl)
            n1435 = Concatenate Strings("cvolume" ("string"), "\r") -> (w2003:string)
            n1436 = VISA Write(VISA resource name=w2004, write buffer=w2003) -> (VISA resource name out=w2014:refnum<visa-resource-name>)  [unwired: 1 in, 2 out]
            n1437 = Concatenate Strings("irun" ("string"), "\r") -> (w2012:string)
            n1438 = VISA Write(VISA resource name=w2014, write buffer=w2012) -> ()  [unwired: 1 in, 3 out]
          }
          frame #1 {
            "Flushing samp" <- TRUE ("Boolean")
          }
        }
      }
      event "Flush Pump 3": Value Change {
        n1439 = event-data() -> ()  [unwired: 7 out]
        n1440 = flat-sequence {
          tunnel: w2024 -> [w2027]
          frame #0 {
            # "set paramaters (rate, volume) for flush, clear volume"
            n1441 = Number To Decimal String(number="Flush rate (uL/m) P3") -> (decimal integer string=w2049:string)  [unwired: 1 in]
            n1442 = local write "Inject Pump 3"(TRUE ("Inject Pump 3")) -> ()
            n1443 = Concatenate Strings("irate  " ("string"), w2049, " u/m" ("string"), "\r") -> (w2051:string)
            n1444 = VISA Write(VISA resource name=w2027, write buffer=w2051) -> (VISA resource name out=w2047:refnum<visa-resource-name>)  [unwired: 1 in, 2 out]
            n1445 = Reciprocal(x="Flush rate (uL/m) P3") -> (1/x=w2031:dbl)
            n1446 = Number To Decimal String(number="Volume (uL) P3") -> (decimal integer string=w2038:string)  [unwired: 1 in]
            n1447 = Multiply(x="Volume (uL) P3", y=w2031) -> (x*y=w2030:dbl)
            n1448 = Concatenate Strings("tvolume  " ("string"), w2038, " u" ("string"), "\r") -> (w2036:string)
            n1449 = Multiply(x=w2030, y=60.0) -> (x*y=→"HP3 Flush Time (s)":dbl)
            n1450 = VISA Write(VISA resource name=w2047, write buffer=w2036) -> (VISA resource name out=w2035:refnum<visa-resource-name>)  [unwired: 1 in, 2 out]
            n1451 = Concatenate Strings("cvolume" ("string"), "\r") -> (w2034:string)
            n1452 = VISA Write(VISA resource name=w2035, write buffer=w2034) -> (VISA resource name out=w2045:refnum<visa-resource-name>)  [unwired: 1 in, 2 out]
            n1453 = Concatenate Strings("irun" ("string"), "\r") -> (w2043:string)
            n1454 = VISA Write(VISA resource name=w2045, write buffer=w2043) -> ()  [unwired: 1 in, 3 out]
          }
          frame #1 {
            "Flushing P3" <- TRUE ("Flushing P3")
          }
        }
      }
      event "Flush Pump 1": Value Change {
        n1455 = event-data() -> ()  [unwired: 7 out]
        n1456 = flat-sequence {
          tunnel: [w2065] -> w2055
          tunnel: w2054 -> [w2058]
          tunnel: w2055 -> [_]
          frame #0 {
            # "set paramaters (rate, volume) for flush, clear volume"
            n1457 = local write "Inject Pump 1"(TRUE ("Inject Pump 1")) -> ()
            n1458 = Number To Decimal String(number="Flush rate (uL/m) P1") -> (decimal integer string=w2081:string)  [unwired: 1 in]
            n1459 = Concatenate Strings("irate  " ("string"), w2081, " u/m" ("string"), "\r") -> (w2083:string)
            n1460 = VISA Write(VISA resource name=w2058, write buffer=w2083) -> (VISA resource name out=w2079:refnum<visa-resource-name>)  [unwired: 1 in, 2 out]
            n1461 = Reciprocal(x="Flush rate (uL/m) P1") -> (1/x=w2062:dbl)
            n1462 = Number To Decimal String(number="Volume (uL) P1") -> (decimal integer string=w2070:string)  [unwired: 1 in]
            n1463 = Multiply(x="Volume (uL) P1", y=w2062) -> (x*y=w2061:dbl)
            n1464 = Concatenate Strings("tvolume  " ("string"), w2070, " u" ("string"), "\r") -> (w2068:string)
            n1465 = Multiply(x=w2061, y=60.0) -> (x*y=→"HP1 Flush Time (s)":dbl)
            n1466 = VISA Write(VISA resource name=w2079, write buffer=w2068) -> (VISA resource name out=w2067:refnum<visa-resource-name>)  [unwired: 1 in, 2 out]
            n1467 = Concatenate Strings("cvolume" ("string"), "\r") -> (w2066:string)
            n1468 = VISA Write(VISA resource name=w2067, write buffer=w2066) -> (VISA resource name out=w2077:refnum<visa-resource-name>)  [unwired: 1 in, 2 out]
            n1469 = Concatenate Strings("irun" ("string"), "\r") -> (w2075:string)
            n1470 = VISA Write(VISA resource name=w2077, write buffer=w2075) -> (VISA resource name out=w2065:refnum<visa-resource-name>)  [unwired: 1 in, 2 out]
          }
          frame #1 {
            "Flushing P1" <- TRUE ("Flushing P3")
          }
        }
      }
      event "Clear Volume": Value Change {
        n1471 = event-data() -> ()  [unwired: 7 out]
        n1472 = Number To Decimal String(number="Normal volume (mL)") -> (decimal integer string=w2090:string)  [unwired: 1 in]
        n1473 = Concatenate Strings("tvolume " ("string"), w2090, " u" ("string"), "\r") -> (w2087:string)
        n1474 = VISA Write(VISA resource name=w2093, write buffer=w2087) -> (VISA resource name out=w2086:refnum<visa-resource-name>)  [unwired: 1 in, 2 out]
        n1475 = local write "Clear Volume"(FALSE ("Clear Volume")) -> ()
        n1476 = Concatenate Strings("cvolume" ("string"), "\r") -> (w2095:string)
        n1477 = VISA Write(VISA resource name=w2086, write buffer=w2095) -> ()  [unwired: 1 in, 3 out]
      }
      event "Clear Volume P3": Value Change {
        n1478 = event-data() -> ()  [unwired: 7 out]
        n1479 = Concatenate Strings("cvolume" ("string"), "\r") -> (w2101:string)
        n1480 = VISA Write(VISA resource name=w2100, write buffer=w2101) -> ()  [unwired: 1 in, 3 out]
        n1481 = local write "Clear Volume P3"(FALSE ("Clear Volume P3")) -> ()
      }
      event "Clear Volume P1": Value Change {
        n1482 = event-data() -> ()  [unwired: 7 out]
        n1483 = Concatenate Strings("cvolume" ("string"), "\r") -> (w2106:string)
        n1484 = local write "Clear Volume P1"(FALSE ("Clear Volume P1")) -> ()
        n1485 = VISA Write(VISA resource name=w2105, write buffer=w2106) -> ()  [unwired: 1 in, 3 out]
      }
      event "Display On P3": Value Change {
        n1486 = event-data() -> ()  [unwired: 7 out]
        n1487 = Select(t="dim 100", s="Display On P3", f="dim 0") -> (s? t:f=w2112:string)
        n1488 = Concatenate Strings(w2112, "\r") -> (w2114:string)
        n1489 = VISA Write(VISA resource name=w2109, write buffer=w2114) -> ()  [unwired: 1 in, 3 out]
      }
      event "Display On P1": Value Change {
        n1490 = event-data() -> ()  [unwired: 7 out]
        n1491 = Select(t="dim 100", s="Display On P1", f="dim 0") -> (s? t:f=w2119:string)
        n1492 = Concatenate Strings(w2119, "\r") -> (w2121:string)
        n1493 = VISA Write(VISA resource name=w2116, write buffer=w2121) -> ()  [unwired: 1 in, 3 out]
      }
      event "Retract Pump 3": Value Change {
        n1494 = event-data() -> ()  [unwired: 7 out]
        n1495 = local write "Retract Pump 3"(FALSE ("Retract Pump 3")) -> ()
        n1496 = case shown="True" "Retract Pump 3" {
          tunnel: w2123 -> [_ w2126]
          frame False {
          }
          frame True {
            n1497 = Number To Decimal String(number="Retract Rate (mL/m)") -> (decimal integer string=w2144:string)  [unwired: 1 in]
            n1498 = Concatenate Strings("wrate  " ("string"), w2144, " u/m" ("string"), "\r") -> (w2146:string)
            n1499 = VISA Write(VISA resource name=w2126, write buffer=w2146) -> (VISA resource name out=w2137:refnum<visa-resource-name>)  [unwired: 1 in, 2 out]
            n1500 = Number To Decimal String(number="Retract Vol 3 (uL)") -> (decimal integer string=w2139:string)  [unwired: 1 in]
            n1501 = Concatenate Strings("tvolume  " ("string"), w2139, " u" ("string"), "\r") -> (w2136:string)
            n1502 = VISA Write(VISA resource name=w2137, write buffer=w2136) -> (VISA resource name out=w2132:refnum<visa-resource-name>)  [unwired: 1 in, 2 out]
            n1503 = Concatenate Strings("cvolume" ("string"), "\r") -> (w2133:string)
            n1504 = VISA Write(VISA resource name=w2132, write buffer=w2133) -> (VISA resource name out=w2127:refnum<visa-resource-name>)  [unwired: 1 in, 2 out]
            n1505 = Concatenate Strings("wrun" ("string"), "\r") -> (w2128:string)
            n1506 = VISA Write(VISA resource name=w2127, write buffer=w2128) -> ()  [unwired: 1 in, 3 out]
          }
        }
      }
      event "Retract Pump 1": Value Change {
        n1507 = event-data() -> ()  [unwired: 7 out]
        n1508 = local write "Retract Pump 1"(FALSE ("Retract Pump 1")) -> ()
        n1509 = case shown="True" "Retract Pump 1" {
          tunnel: w2148 -> [_ w2153]
          frame False {
          }
          frame True {
            n1510 = local read "Retract Rate (mL/m)"() -> (w2151:dbl)
            n1511 = Number To Decimal String(number=w2151) -> (decimal integer string=w2169:string)  [unwired: 1 in]
            n1512 = Concatenate Strings("wrate  " ("string"), w2169, " u/m" ("string"), "\r") -> (w2171:string)
            n1513 = VISA Write(VISA resource name=w2153, write buffer=w2171) -> (VISA resource name out=w2163:refnum<visa-resource-name>)  [unwired: 1 in, 2 out]
            n1514 = Number To Decimal String(number="Retract Vol 1 (uL)") -> (decimal integer string=w2165:string)  [unwired: 1 in]
            n1515 = Concatenate Strings("tvolume  " ("string"), w2165, " u" ("string"), "\r") -> (w2162:string)
            n1516 = VISA Write(VISA resource name=w2163, write buffer=w2162) -> (VISA resource name out=w2159:refnum<visa-resource-name>)  [unwired: 1 in, 2 out]
            n1517 = Concatenate Strings("cvolume" ("string"), "\r") -> (w2160:string)
            n1518 = VISA Write(VISA resource name=w2159, write buffer=w2160) -> (VISA resource name out=w2154:refnum<visa-resource-name>)  [unwired: 1 in, 2 out]
            n1519 = Concatenate Strings("wrun" ("string"), "\r") -> (w2155:string)
            n1520 = VISA Write(VISA resource name=w2154, write buffer=w2155) -> ()  [unwired: 1 in, 3 out]
          }
        }
      }
      event "Flip Green Filter": Value Change {
        n1521 = event-data() -> ()  [unwired: 7 out]
        n1522 = Not(x="Flip Green Filter") -> (.not. x?=w2173:bool)
        n1523 = local write "Flip Green Filter"(w2173) -> ()
        n1524 = flat-sequence {
          tunnel: w2181 -> [w2186]
          tunnel: w2180 -> [w2185]
          tunnel: [w2183] -> w2178
          tunnel: [w2182] -> w2177
          tunnel: [w2188] -> w2176
          tunnel: w2178 -> [w2188]
          tunnel: [w2187] -> w2175
          tunnel: w2177 -> [w2187]
          tunnel: w2176 -> [w2192]
          tunnel: w2175 -> [w2191]
          tunnel: [w2190] -> w2179
          frame #0 {
            n1525 = xnode "Read/Write Control"("FPGA VI Reference In"=w2186, "error in"=w2185, "Green Filter Flipper"=TRUE) -> ("FPGA VI Reference Out"=w2183:T20, "error out"=w2182:errorcluster)
          }
          frame #1 {
            n1526 = Wait (ms)(milliseconds to wait=u32 100) -> ()  [unwired: 1 out]
          }
          frame #2 {
            n1527 = xnode "Read/Write Control"("FPGA VI Reference In"=w2192, "error in"=w2191, "Green Filter Flipper"=FALSE) -> ("error out"=w2190:errorcluster)  [unwired: 1 out]
          }
        }
      }
      event "Pump 1 contents", "Pump 3 contents": Value Change {
        n1528 = event-data() -> ()  [unwired: 7 out]
        n1529 = local read "Pump 1 contents"() -> (→"Pump 1 cont disp":string)
        n1530 = local read "Pump 3 contents"() -> (→"Pump 3 cont disp":string)
      }
      event "Reset Trap Pos. FB": Value Change {
        n1531 = event-data() -> ()  [unwired: 7 out]
        n1532 = xnode "Read/Write Control"("FPGA VI Reference In"=w2198, "error in"=w2197, "Trap Pos. FB Reset"="Reset Trap Pos. FB") -> ()  [unwired: 2 out]
      }
      event "Rem fb disp offset": Value Change {
        n1533 = event-data() -> ()  [unwired: 7 out]
        n1534 = local write "Rem fb disp offset"(FALSE ("Rem fb disp offset")) -> ()
        n1535 = local read "Mean T1 Position (nm)"() -> (w2200:dbl)
        n1536 = local read "FB Trap Pos Offset"() -> (w2201:dbl)
        n1537 = Subtract(x=w2201, y=w2200) -> (x-y=w2199:dbl)
        n1538 = local write "FB Trap Pos Offset"(w2199) -> ()
      }
      event "Threshold (nm)": Value Change {
        n1539 = event-data() -> ()  [unwired: 7 out]
        n1540 = flat-sequence {
          tunnel: w2205 -> [w2213]
          tunnel: w2204 -> [w2212]
          tunnel: [w2206] -> w2203
          tunnel: w2203 -> [w2219]
          frame #0 {
            n1541 = xnode "Read/Write Control"("FPGA VI Reference In"=w2213, "error in"=w2212) -> ("FPGA VI Reference Out"=w2209:T20, "error out"=w2208:errorcluster, "FPGA TTrig Thresh"=w2210:i64)
            n1542 = local read "Threshold stored (nm)"() -> (w2218:dbl)
            n1543 = local read "Threshold (nm)"() -> (w2206:dbl)
            n1544 = local read "AOM X Cal (nm/MHz)"() -> (w2216:dbl)
            n1545 = Subtract(x=w2206, y=w2218) -> (x-y=w2217:dbl)
            n1546 = Divide(x=w2217, y=w2216) -> (x/y=w2214:dbl)
